vi "push_to_grab_image.vi"(8 "Boolean 2":bool, 9 "stop 2":bool) -> (2 "Numeric 2":i32)   [LabVIEW 2015]
uses:
  <vilib>/userdefined/High Color/IMAQdx.ctl
  <vilib>/vision/driver/NI_Vision_Acquisition_Software.lvlib
panel:
  in  "Numeric":i32
  out "Image":T1(plugin-control)
  in  "Boolean":bool
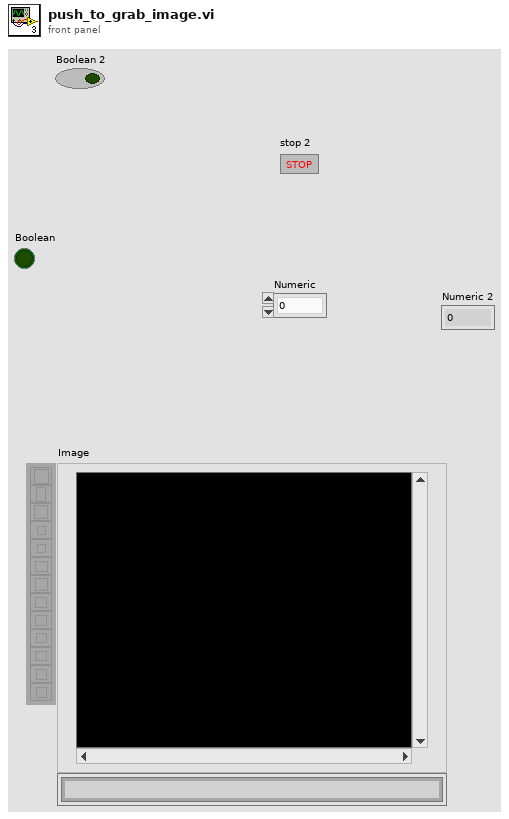
[diagram p1: front panel]
types:
  T1 = typedef "IMAQ Image.ctl" = refnum<image>
  T2 = typedef "IMAQdx.ctl" = refnum<k21>
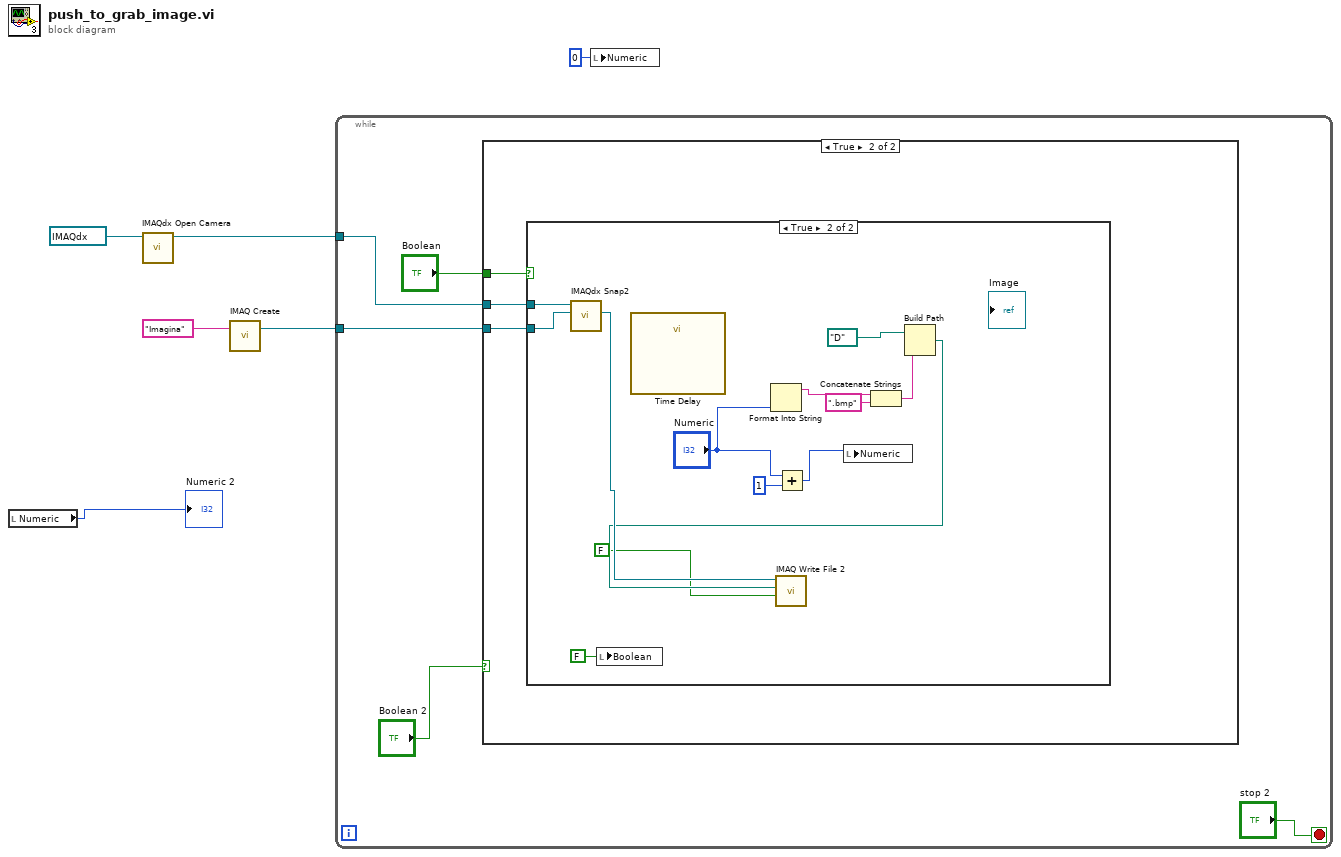
[diagram p0: block diagram]
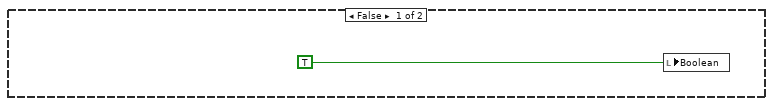
[diagram p2: hidden frame]
diagram:
  n1 = local read "Numeric"() -> (→"Numeric 2":i32)
  n2 = call <vilib>:"IMAQdx Open Camera.vi"("Session In"=T2 "cam0") -> ("Session Out"=w4:T2)  [unwired: 9 in, 1 out]
  n3 = call "IMAQ Create"("Image Name"="Imagina") -> ("New Image"=w3:T1)  [unwired: 4 in, 1 out]
  n4 = while {
    tunnel: w4 -> [w9]
    tunnel: w3 -> [w8]
    stop <- "stop 2" stop-if-true
    n5 = case shown="True" "Boolean 2" {
      tunnel: "Boolean" -> [_ w15]
      tunnel: w9 -> [_ w14]
      tunnel: w8 -> [_ w13]
      frame False {
        n6 = local write "Boolean"(TRUE) -> ()
      }
      frame True {
        n7 = case shown="True" w15 {
          tunnel: w14 -> [_ w27]
          tunnel: w13 -> [_ w26]
          frame False {
          }
          frame True {
            n8 = call <vilib>:"IMAQdx Snap2.vi"("Image In"=w26, "Session In"=w27) -> ("Image Out"=w21:T1)  [unwired: 7 in, 2 out]
            n9 = local write "Boolean"(FALSE) -> ()
            n10 = call "Time Delay"() -> ()  [unwired: 11 in, 1 out]
            n11 = Format Into String("Numeric") -> (resulting string=w24:string)  [unwired: 3 in, 1 out]
            n12 = Add(x="Numeric", y=1) -> (x+y=w17:i32)
            n13 = local write "Numeric"(w17) -> ()
            n14 = Concatenate Strings(w24, ".bmp" ("string")) -> (w22:string)
            n15 = Build Path(base path=path "D:/", name or relative path=w22) -> (appended path=w20:path)
            n16 = call-poly "IMAQ Write File 2"("Compress? (N)"=FALSE, "File Path"=w20, "Image"=w21) -> ()  [unwired: 7 in, 2 out]
          }
        }
      }
    }
  }
  n17 = local write "Numeric"(0 ("Numeric")) -> ()
